vi "Config Delete Section.vi"(7 "Section Name":string, 8 "error in":errorcluster, 11 "Config Cluster in":T1) -> (0 "error out":errorcluster, 2 "Found?":bool, 3 "Config Cluster out":T1)   [LabVIEW 2017]
uses:
  Config Cluster.ctl
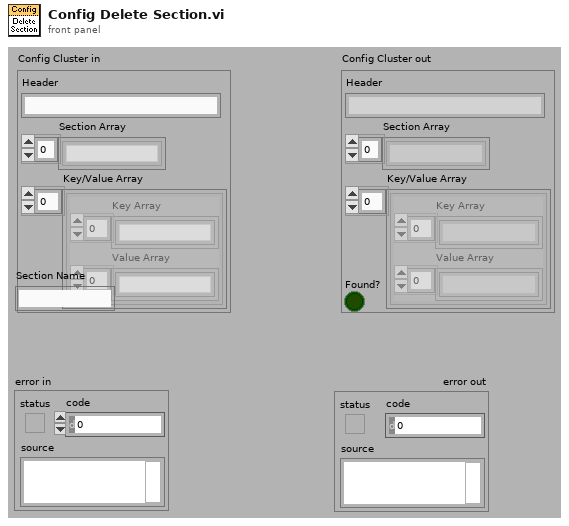
[diagram p1: front panel]
types:
  T1 = typedef "Config Cluster.ctl" = cluster{"Header":string, "Section Array":string[], "Key/Value Array":cluster{"Key Array":string[], "Value Array":string[]}[]}
  T2 = cluster{"Key Array":string[], "Value Array":string[]}[]
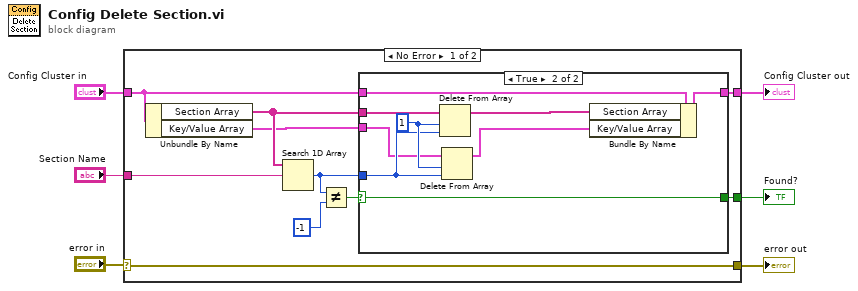
[diagram p0: block diagram]
diagram:
  n1 = case shown="No Error" "error in" {
    selector: "error in" -> [w8 w29]
    tunnel: [w8 w29] -> w5
    tunnel: "Config Cluster in" -> [w13 w28]
    tunnel: [w9 w28] -> w3
    tunnel: "Section Name" -> [w16 _]
    tunnel: [w7 _] -> w1
    frame No Error {
      n2 = Unbundle By Name(w13) -> ("Section Array"=w11:string[], "Key/Value Array"=w10:T2)
      n3 = Search 1D Array(1D array=w11, element=w16) -> (index of element=w12:i32)  [unwired: 1 in]
      n4 = Not Equal?(x=w12, y=-1) -> (x != y?=w14:bool)
      n5 = case shown="True" w14 {
        selector: w14 -> [w17 w19]
        tunnel: w13 -> [w18 w21]
        tunnel: w12 -> [_ w25]
        tunnel: w11 -> [_ w27]
        tunnel: w10 -> [_ w24]
        tunnel: [w18 w20] -> w9
        tunnel: [w17 w19] -> w7
        frame False {
          # "Section not found, nothing is deleted, Found? = F."
        }
        frame True {
          w26 = 1
          n6 = Delete From Array(array=w27, length=w26, index=w25) -> (array with subset deleted=w23:string[])  [unwired: 1 out]
          n7 = Delete From Array(array=w24, length=w26, index=w25) -> (array with subset deleted=w22:T2)  [unwired: 1 out]
          n8 = Bundle By Name(cluster=w21, "Section Array"=w23, "Key/Value Array"=w22) -> (w20:T1)
        }
      }
    }
    frame Error {
    }
  }
  "error out" <- w5
  "Config Cluster out" <- w3
  "Found?" <- w1
